vi "red_tweezers_globals.vi"() -> ()   [LabVIEW 2019]
doc: "This global variable can be used to remote-control Red Tweezers as well as to read out what it's doing. You must always ensure that the spots and selection arrays are the same length!\n\n\n(the line below ensures settings are saved)\n[Red Tweezers Save Settings]"
uses:
  spot.ctl
  line_trapping.ctl
  selection_element.ctl
panel:
  in  "Selection/Group":T1[](array[typedef])
  in  "Spots":T2[](array[typedef]) {"Amplitude Correction" step=0.1; "Line Trapping"."Phase Gradient" step=0.05; "Line Trapping"."Vector"."x" step=1e-06 format="%#_6p"; "Line Trapping"."Vector"."y" step=1e-06 format="%#_6p"; "Line Trapping"."Vector"."z" step=1e-06 format="%#_6p"; "NA Position"."r" step=1e-06; "NA Position"."y" step=1e-06; "NA Position"."x" step=1e-06; "Position"."z" step=1e-06; "Position"."y" step=1e-06; "Position"."x" step=1e-06; "Phase" step=0.7753; "Intensity" step=0.1}
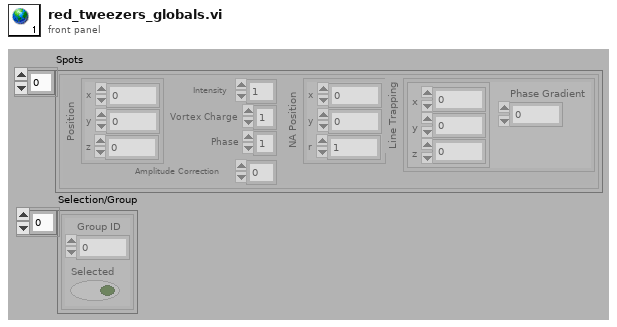
[diagram p1: front panel]
types:
  T1 = typedef "selection_element.ctl" = cluster{"Group ID":i32, "Selected":bool}
  T2 = typedef "spot.ctl" = cluster{"Position":cluster{"x":dbl, "y":dbl, "z":dbl}, "Intensity":dbl, "Vortex Charge":i8, "Phase":dbl, "NA Position":cluster{"x":dbl, "y":dbl, "r":dbl}, "Line Trapping":T3, "Amplitude Correction":dbl}
  T3 = typedef "line_trapping.ctl" = cluster{"Vector":cluster{"x":dbl, "y":dbl, "z":dbl}, "Phase Gradient":dbl}
diagram:
